vi "OPP.Mixer.vi"() -> ()   [LabVIEW 2020]
uses:
  Controls/MixerSlider/MixerSlider.xctl
  Typedefs/Mixer.Channel Property Data.ctl
  SubVIs/Mixer.Globals.vi
panel:
  in  "TTS":dbl(xcontrol)
  in  "Tester":dbl(xcontrol) caption="Waver mic"
  in  "Video":dbl(xcontrol)
  in  "Participant":dbl(xcontrol) caption="Stimulus"
  in  "Mic":dbl(xcontrol) caption="Talkback"
  in  "Waver":dbl(xcontrol) caption="Stimulus"
  in  "Caregiver":dbl(xcontrol) caption="Stimulus"
  # "A: Caregiver"
  # "B: Waver"
  # "C: Participant"
  # "D: Tester"
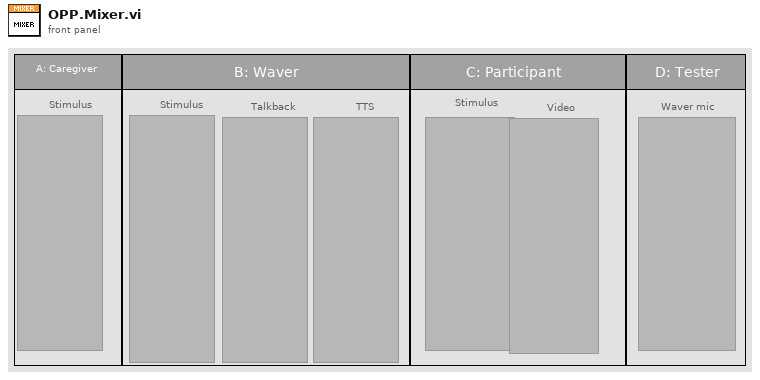
[diagram p1: front panel]
types:
  T1 = enum8{"Enabled", "Disabled", "Disabled and Grayed Out"}
  T2 = typedef "Mixer.Channel Property Data.ctl" = cluster{"channel":string, "property":string, "value":bool}
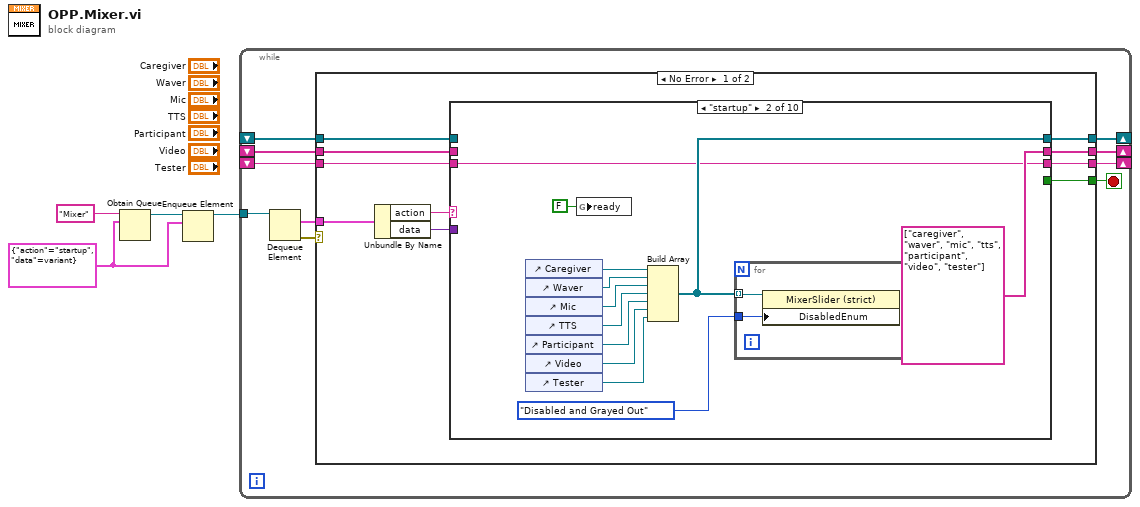
[diagram p0: block diagram]
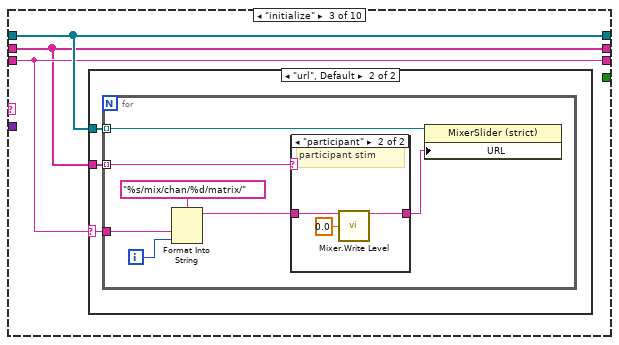
[diagram p3: hidden frame]
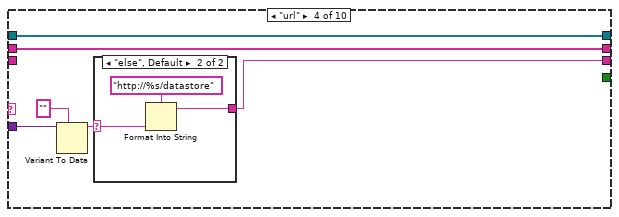
[diagram p6: hidden frame]
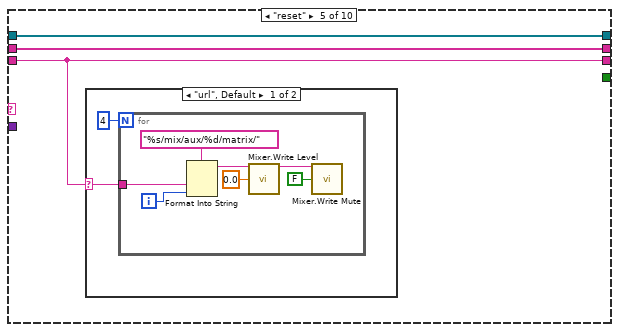
[diagram p8: hidden frame]
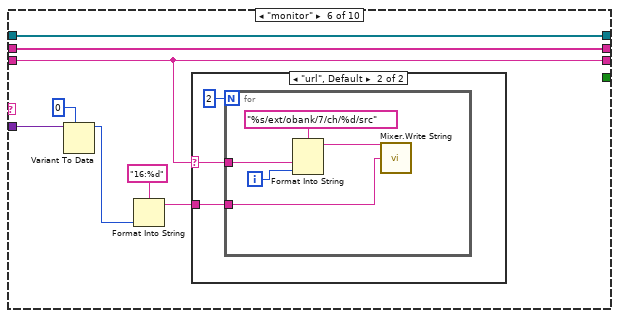
[diagram p10: hidden frame]
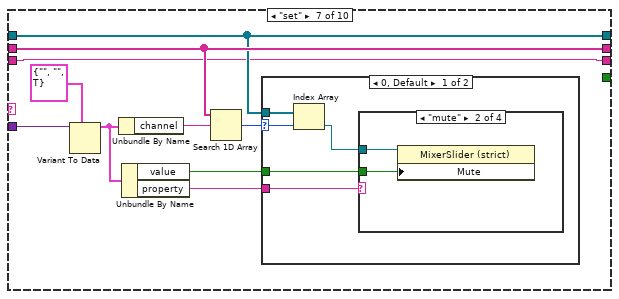
[diagram p12: hidden frame]
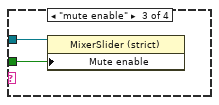
[diagram p14: hidden frame]
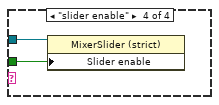
[diagram p15: hidden frame]
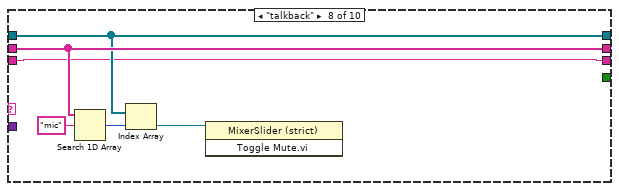
[diagram p17: hidden frame]
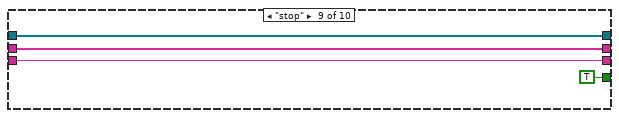
[diagram p18: hidden frame]
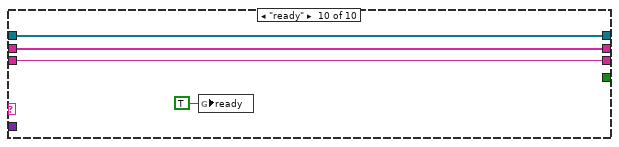
[diagram p19: hidden frame]
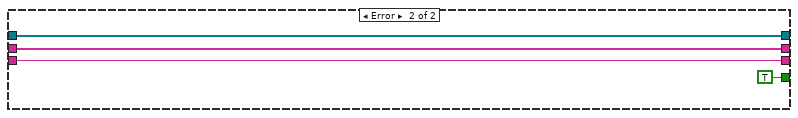
[diagram p20: hidden frame]
diagram:
  w1 = cluster{"action":string, "data":variant} {"action"="startup", "data"=variant}
  n1 = Obtain Queue(name (unnamed)="Mixer", element data type=w1) -> (queue out=w2:refnum<queue>)  [unwired: 3 in, 2 out]
  n2 = Enqueue Element(queue=w2, element=w1) -> (queue out=w3:refnum<queue>)  [unwired: 2 in, 2 out]
  n3 = while {
    tunnel: w3 -> [w14]
    shift-right: [w11] -> _
    shift-left: _ -> [w10]
    shift-right: [w8] -> _
    shift-left: _ -> [w7]
    shift-right: [w6] -> _
    shift-left: _ -> [w5]
    stop <- w9 stop-if-true
    n4 = Dequeue Element(queue=w14) -> (element=w12:cluster{"action":string, "data":variant}, error out=w13:errorcluster)  [unwired: 2 in, 2 out]
    n5 = case shown="No Error" w13 {
      tunnel: w12 -> [w24 _]
      tunnel: [w21 w135] -> w11
      tunnel: w10 -> [w20 w135]
      tunnel: [w19 TRUE] -> w9
      tunnel: [w18 w133] -> w8
      tunnel: w7 -> [w17 w133]
      tunnel: [w16 w132] -> w6
      tunnel: w5 -> [w15 w132]
      frame No Error {
        n6 = Unbundle By Name(w24) -> ("action"=w23:string, "data"=w22:variant)
        n7 = case shown="\"startup\"" w23 {
          tunnel: w22 -> [_ _ _ w64 _ w85 w106 _ _ _]
          tunnel: [w27 w38 w44 w62 w71 w88 w100 w121 w127 w131] -> w21
          tunnel: w20 -> [w27 _ w44 w62 w71 w88 w100 w121 w127 w131]
          tunnel: [_ _ _ _ _ _ _ _ TRUE _] -> w19
          tunnel: [w26 string[] ["caregiver", "waver", "mic", "tts", "participant", "video", "tester"] w42 w60 w70 w87 w104 w123 w125 w130] -> w18
          tunnel: w17 -> [w26 _ w42 w60 w70 w87 w104 w123 w125 w130]
          tunnel: [w25 w31 w43 w59 w69 w86 w97 w120 w124 w129] -> w16
          tunnel: w15 -> [w25 w31 w43 _ w69 w86 w97 w120 w124 w129]
          frame "", Default {
          }
          frame "startup" {
            n8 = control-ref of="Caregiver"() -> (w39:refnum<vi>)
            n9 = control-ref of="Waver"() -> (w35:refnum<vi>)
            n10 = control-ref of="Mic"() -> (w34:refnum<vi>)
            n11 = control-ref of="TTS"() -> (w28:refnum<vi>)
            n12 = control-ref of="Participant"() -> (w33:refnum<vi>)
            n13 = control-ref of="Video"() -> (w32:refnum<vi>)
            n14 = control-ref of="Tester"() -> (w29:refnum<vi>)
            n15 = global write "Mixer.Globals.vi" "ready"(FALSE ("ready")) -> ()
            n16 = Build Array(w39, w35, w34, w28, w33, w32, w29) -> (w38:refnum<vi>[])
            n17 = for {
              tunnel: w38 -> [w41] mode=indexing
              tunnel: T1."Disabled and Grayed Out" ("Disabled") -> [w40]
              n18 = property class="MixerSlider (strict)"(reference=w41, "DisabledEnum"=w40) -> ()  [unwired: 1 in, 2 out]
            }
          }
          frame "initialize" {
            n19 = case shown="\"url\", Default" w43 {
              selector: w43 -> [_ w46]
              tunnel: w44 -> [_ w47]
              tunnel: w42 -> [_ w45]
              frame "test" {
              }
              frame "url", Default {
                n20 = for {
                  tunnel: w47 -> [w54] mode=indexing
                  tunnel: w46 -> [w49]
                  tunnel: w45 -> [w48] mode=indexing
                  i -> [w50]
                  n21 = Format Into String(format string="%s/mix/chan/%d/matrix/", w49, w50) -> (resulting string=w52:string)  [unwired: 2 in, 1 out]
                  n22 = case shown="\"participant\"" w48 {
                    tunnel: w52 -> [w55 w58]
                    tunnel: [w55 w57] -> w51
                    frame "0", Default {
                    }
                    frame "participant" {
                      # "participant stim"
                      n23 = call "Mixer.Write Level.vi"("baseURL"=w58, "value"=0.0) -> ("baseURL out"=w57:string)  [unwired: 12 in, 1 out]
                    }
                  }
                  n24 = property class="MixerSlider (strict)"(reference=w54, "URL"=w51) -> ()  [unwired: 1 in, 2 out]
                }
              }
            }
          }
          frame "url" {
            n25 = Variant To Data(type="", Variant=w64) -> (data=w61:string)  [unwired: 1 in, 1 out]
            n26 = case shown="\"else\", Default" w61 {
              selector: w61 -> [w65 w68]
              tunnel: [w65 w66] -> w59
              frame "test" {
              }
              frame "else", Default {
                n27 = Format Into String(format string="http://%s/datastore", w68) -> (resulting string=w66:string)  [unwired: 2 in, 1 out]
              }
            }
          }
          frame "reset" {
            n28 = case shown="\"url\", Default" w69 {
              selector: w69 -> [w72 _]
              frame "url", Default {
                n29 = for {
                  N: 4 -> [_]
                  tunnel: w72 -> [w80]
                  i -> [w79]
                  n30 = Format Into String(format string="%s/mix/aux/%d/matrix/", w80, w79) -> (resulting string=w78:string)  [unwired: 2 in, 1 out]
                  n31 = call "Mixer.Write Level.vi"("baseURL"=w78, "value"=0.0) -> ("baseURL out"=w76:string)  [unwired: 12 in, 1 out]
                  n32 = call "Mixer.Write Mute.vi"("baseURL"=w76, "mute"=FALSE) -> ()  [unwired: 13 in, 1 out]
                }
              }
              frame "test" {
              }
            }
          }
          frame "monitor" {
            n33 = Variant To Data(type=0, Variant=w85) -> (data=w82:i32)  [unwired: 1 in, 1 out]
            n34 = Format Into String(format string="16:%d", w82) -> (resulting string=w81:string)  [unwired: 2 in, 1 out]
            n35 = case shown="\"url\", Default" w86 {
              selector: w86 -> [_ w90]
              tunnel: w81 -> [_ w89]
              frame "test" {
              }
              frame "url", Default {
                n36 = for {
                  N: 2 -> [_]
                  tunnel: w90 -> [w96]
                  tunnel: w89 -> [w92]
                  i -> [w95]
                  n37 = Format Into String(format string="%s/ext/obank/7/ch/%d/src", w96, w95) -> (resulting string=w93:string)  [unwired: 2 in, 1 out]
                  n38 = call "Mixer.Write String.vi"("url"=w93, "value"=w92) -> ()  [unwired: 13 in, 1 out]
                }
              }
            }
          }
          frame "set" {
            n39 = Variant To Data(type=T2 {"channel"="", "property"="", "value"=TRUE} ("Cluster"), Variant=w106) -> (data=w101:T2)  [unwired: 1 in, 1 out]
            n40 = Unbundle By Name(w101) -> ("channel"=w103:string)
            n41 = Unbundle By Name(w101) -> ("value"=w98:bool, "property"=w99:string)
            n42 = Search 1D Array(1D array=w104, element=w103) -> (index of element=w102:i32)  [unwired: 1 in]
            n43 = case shown="0, Default" w102 {
              selector: w102 -> [w111 _]
              tunnel: w100 -> [w110 _]
              tunnel: w99 -> [w109 _]
              tunnel: w98 -> [w107 _]
              frame 0, Default {
                n44 = Index Array(array=w110, index=w111) -> (element=w108:refnum<vi>)
                n45 = case shown="\"mute\"" w109 {
                  tunnel: w108 -> [_ w113 w115 w117]
                  tunnel: w107 -> [_ w112 w114 w116]
                  frame "", Default {
                  }
                  frame "mute" {
                    n46 = property class="MixerSlider (strict)"(reference=w113, "Mute"=w112) -> ()  [unwired: 1 in, 2 out]
                  }
                  frame "mute enable" {
                    n47 = property class="MixerSlider (strict)"(reference=w115, "Mute enable"=w114) -> ()  [unwired: 1 in, 2 out]
                  }
                  frame "slider enable" {
                    n48 = property class="MixerSlider (strict)"(reference=w117, "Slider enable"=w116) -> ()  [unwired: 1 in, 2 out]
                  }
                }
              }
              frame -1 {
              }
            }
          }
          frame "talkback" {
            n49 = Search 1D Array(1D array=w123, element="mic") -> (index of element=w122:i32)  [unwired: 1 in]
            n50 = Index Array(array=w121, index=w122) -> (element=w118:refnum<vi>)
            n51 = invoke class="MixerSlider (strict)" method="Toggle Mute.vi"(reference=w118) -> ()  [unwired: 2 in, 3 out]
          }
          frame "stop" {
          }
          frame "ready" {
            n52 = global write "Mixer.Globals.vi" "ready"(TRUE ("ready")) -> ()
          }
        }
      }
      frame Error {
      }
    }
  }
